vi "PXI-Enumerate Devices.vi"(11 "error in (no error)":errorcluster) -> (4 "Devices":T1[](array[typedef]), 15 "error out":errorcluster)   [LabVIEW 2020]
uses:
  Typedefs/PXI-Device Spec.ctl
  <resource>/objmgr/daqmx.rc
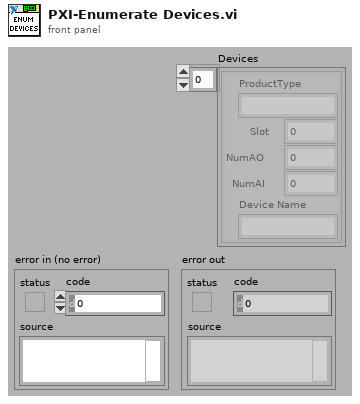
[diagram p1: front panel]
types:
  T1 = typedef "PXI-Device Spec.ctl" = cluster{"Slot":i32, "ProductType":string, "NumAO":i32, "NumAI":i32, "Device Name":string}
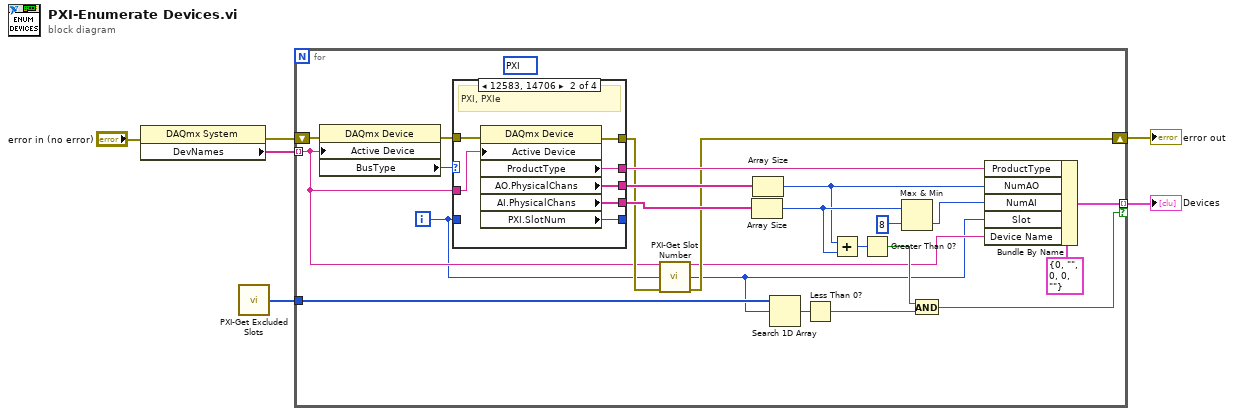
[diagram p0: block diagram]
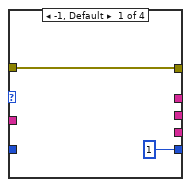
[diagram p2: hidden frame]
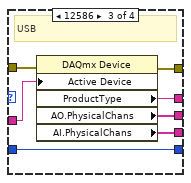
[diagram p3: hidden frame]
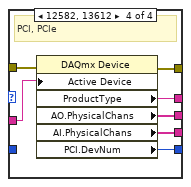
[diagram p4: hidden frame]
diagram:
  n1 = property class="DAQmx System"(error in="error in (no error)") -> (error out=w4:errorcluster, "DevNames"=w3:tag[])  [unwired: 1 in, 1 out]
  n2 = call "PXI-Get Excluded Slots.vi"() -> ("excluded slots"=w6:i32[])  [unwired: 14 in, 1 out]
  n3 = for {
    tunnel: w3 -> [w10] mode=indexing
    shift-right: [w11] -> w5
    shift-left: w4 -> [w29]
    tunnel: w6 -> [w30]
    tunnel: [w16] -> w1 mode=indexing if=w13
    i -> [w7]
    (unwired) 12583 items=["PCI"=12582, "PCIe"=13612, "PXI"=12583, "PXIe"=14706, "SCXI"=12584, "SCC"=14707, "PCCard"=12585, "USB"=12586, "CompactDAQ"=14637, "TCP/IP"=14828, "Unknown"=12588, "SwitchBlock"=15870] ("BusType")
    n4 = property class="DAQmx Device"(error in=w29, "Active Device"=w10) -> (error out=w28:errorcluster, "BusType"=w27:i32)  [unwired: 1 in, 1 out]
    n5 = case shown="12583, 14706" w27 {
      tunnel: [_ w39 w46 w53] -> w26
      tunnel: [_ w38 w45 w52] -> w25
      tunnel: [w32 w37 w44 w51] -> w12
      tunnel: [u32 1 ("PCI.DevNum") w36 w41 w50] -> _
      tunnel: w28 -> [w32 w35 w43 w49]
      tunnel: w10 -> [_ w34 w42 w48]
      tunnel: w7 -> [_ _ w41 _]
      tunnel: [_ w33 w40 w47] -> w20
      frame -1, Default {
      }
      frame 12583, 14706 {
        # "PXI, PXIe"
        n6 = property class="DAQmx Device"(error in=w35, "Active Device"=w34) -> (error out=w37:errorcluster, "ProductType"=w33:string, "AO.PhysicalChans"=w39:tag[], "AI.PhysicalChans"=w38:tag[], "PXI.SlotNum"=w36:u32)  [unwired: 1 in, 1 out]
      }
      frame 12586 {
        # "USB"
        n7 = property class="DAQmx Device"(error in=w43, "Active Device"=w42) -> (error out=w44:errorcluster, "ProductType"=w40:string, "AO.PhysicalChans"=w46:tag[], "AI.PhysicalChans"=w45:tag[])  [unwired: 1 in, 1 out]
      }
      frame 12582, 13612 {
        # "PCI, PCIe"
        n8 = property class="DAQmx Device"(error in=w49, "Active Device"=w48) -> (error out=w51:errorcluster, "ProductType"=w47:string, "AO.PhysicalChans"=w53:tag[], "AI.PhysicalChans"=w52:tag[], "PCI.DevNum"=w50:u32)  [unwired: 1 in, 1 out]
      }
    }
    n9 = call "PXI-Get Slot Number.vi"("DAQmx Device Name in"=w10, "Index"=w7, "error in (no error)"=w12) -> ("DAQmx Device Name out"=w9:tag, "Slot num"=w8:i32, "error out"=w11:errorcluster)  [unwired: 10 in]
    n10 = Array Size(array=w25) -> (size(s)=w19:i32)
    n11 = Array Size(array=w26) -> (size(s)=w18:i32)
    n12 = Search 1D Array(1D array=w30, element=w8) -> (index of element=w23:i32)  [unwired: 1 in]
    n13 = Less Than 0?(x=w23) -> (x < 0?=w15:bool)
    n14 = Add(x=w18, y=w19) -> (x+y=w24:i32)
    n15 = Greater Than 0?(x=w24) -> (x > 0?=w14:bool)
    n16 = Max & Min(x=w19, y=8) -> (min(x,y)=w17:i32)  [unwired: 1 out]
    n17 = And(x=w14, y=w15) -> (x .and. y?=w13:bool)
    n18 = Bundle By Name(cluster=T1 {"Slot"=0, "ProductType"="", "NumAO"=0, "NumAI"=0, "Device Name"=""} ("Device"), "ProductType"=w20, "NumAO"=w18, "NumAI"=w17, "Slot"=w8, "Device Name"=w9) -> (w16:T1)
  }
  "error out" <- w5
  "Devices" <- w1
